vi "IMRP.vi"() -> ()   [LabVIEW 2015]
uses:
  <vilib>/vision/Instrument.llb/Barcode Search Options.ctl
  <vilib>/vision/NI_Vision_Development_Module.lvlib
panel:
  out "String 2":string
  out "String":string
  out "x = y?":bool[](array[boolean])
  out "Barcode Read 2":cluster{"Data":string, "Barcode Type":string}[](array[cluster])
  in  "Delay (s.) 2":dbl(slide)=0.4897959183673469 scale=0.0..2.0
  in  "Stop":bool
  in  "Delay (s.)":dbl(slide)=0.4897959183673469 scale=0.0..2.0
  out "Image":T1(plugin-control)
  out "Number of Barcodes Found":u32
  out "Barcode Read":cluster{"Data":string, "Barcode Type":string}[](array[cluster])
  out "Barcode ANSI/CEN/ISO Grading Report":T2(array[cluster])
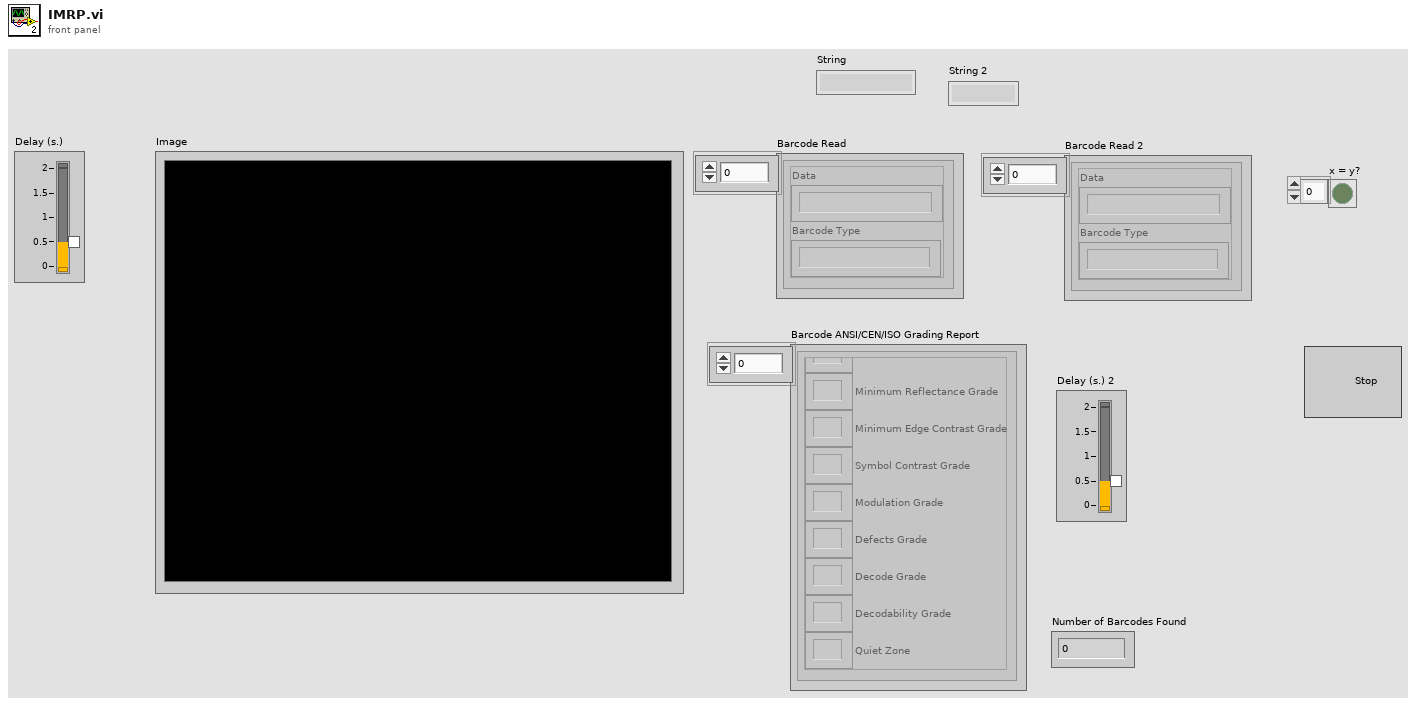
[diagram p1: front panel]
types:
  T1 = typedef "IMAQ Image.ctl" = refnum<image>
  T2 = cluster{"Overall Grade":string, "Edge Determination Grade":string, "Minimum Reflectance Grade":string, "Minimum Edge Contrast Grade":string, "Symbol Contrast Grade":string, "Modulation Grade":string, "Defects Grade":string, "Decode Grade":string, "Decodability Grade":string, "Quiet Zone":string}[]
  T3 = typedef "Barcode Search Options.ctl" = cluster{"Min Bar Width":u32, "Min Edge Strength":u32, "Min Bars":u32, "Skip Location Search?":bool}
  T4 = cluster{"Calculate Grading Report":bool, "Scan Width ":i32}
  T5 = cluster{"Data":string, "Special Char 1":string, "Special Char 2":string, "Checksum(s)":string, "Barcode Type":u32, "Confidence Level":sgl, "Bounding Box":cluster{"x":sgl, "y":sgl}[]}[]
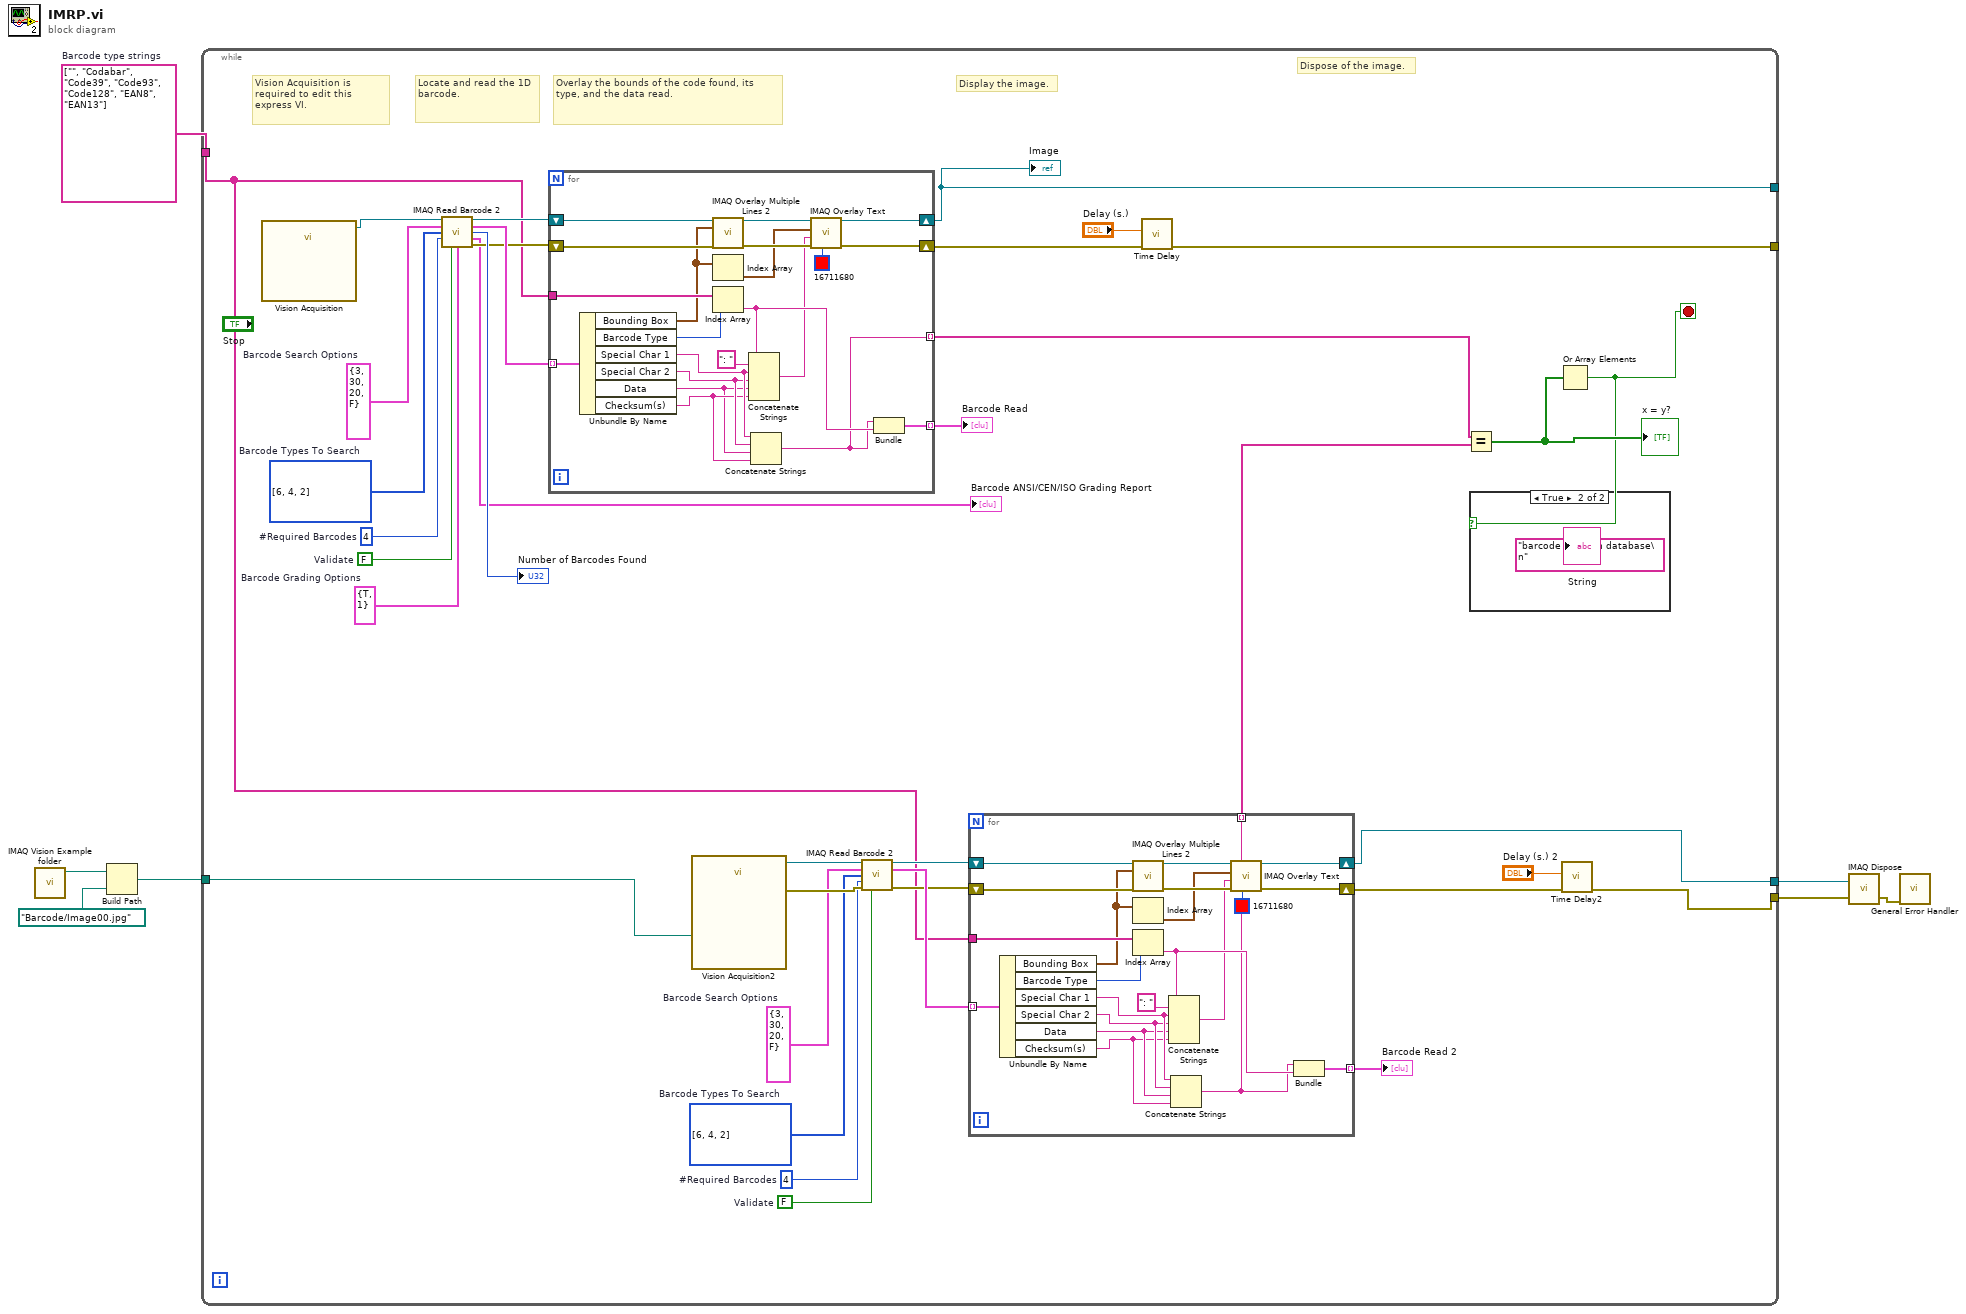
[diagram p0: block diagram]
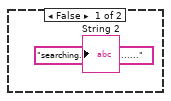
[diagram p2: hidden frame]
diagram:
  w7 = string[] ["", "Codabar", "Code39", "Code93", "Code128", "EAN8", "EAN13"]  # Barcode type strings
  # "Dispose of the image."
  n1 = call "IMAQ Vision Example folder.vi"() -> ("Example Image Path"=w6:path)  [unwired: 11 in]
  n2 = Build Path(base path=w6, name or relative path=path "Barcode/Image00.jpg" ("appended path")) -> (appended path=w4:path)
  n3 = while {
    tunnel: [w35] -> _
    tunnel: [w29] -> _
    tunnel: w7 -> [w15]
    tunnel: w4 -> [w14]
    tunnel: [w13] -> w2
    tunnel: [w12] -> w1
    stop <- w8 stop-if-true
    w17 = T3 {"Min Bar Width"=3, "Min Edge Strength"=30, "Min Bars"=20, "Skip Location Search?"=FALSE}  # Barcode Search Options
    w26 = u32 4  # #Required Barcodes
    w22 = u32[] [6, 4, 2] items=["Reserved", "Codabar", "Code 39", "Code 93", "Code 128", "EAN 8", "EAN 13", "Interleaved 2 of 5", "MSI", "UPCA", "Pharmacode", "RSS Limited"]  # Barcode Types To Search
    w18 = FALSE  # Validate
    w32 = T4 {"Calculate Grading Report"=TRUE, "Scan Width "=1}  # Barcode Grading Options
    w33 = T3 {"Min Bar Width"=3, "Min Edge Strength"=30, "Min Bars"=20, "Skip Location Search?"=FALSE}  # Barcode Search Options
    w43 = u32 4  # #Required Barcodes
    w39 = u32[] [6, 4, 2] items=["Reserved", "Codabar", "Code 39", "Code 93", "Code 128", "EAN 8", "EAN 13", "Interleaved 2 of 5", "MSI", "UPCA", "Pharmacode", "RSS Limited"]  # Barcode Types To Search
    w34 = FALSE  # Validate
    # "Display the image."
    # "Locate and read the 1D barcode."
    # "Vision Acquisition is required to edit this express VI."
    # "Overlay the bounds of the code found, its type, and the data read."
    n4 = call "Vision Acquisition"() -> ("Image Out"=w28:T1)  [unwired: 26 in, 1 out]
    n5 = call "IMAQ Read Barcode 2"("Image"=w28, "Barcode Search Options"=w33, "Barcode Types To Search"=w39, "Num of Required Barcodes"=w43, "Validate"=w34, "Barcode Grading Options"=w32) -> ("Image (duplicate)"=w41:T1, "Barcodes"=w42:T5, "Num of Barcodes"=→"Number of Barcodes Found":u32, "Barcode ANSI/CEN/ISO Grading Report"=→"Barcode ANSI/CEN/ISO Grading Report":T2, "error out"=w38:errorcluster)  [unwired: 5 in]
    n6 = for {
      tunnel: w42 -> [w87] mode=indexing
      tunnel: w15 -> [w86]
      shift-right: [w82] -> w35
      shift-left: w41 -> [w78]
      shift-right: [w79] -> w37
      shift-left: w38 -> [w81]
      tunnel: [w74] -> w31 mode=indexing
      tunnel: [w67] -> w11 mode=indexing
      n7 = Unbundle By Name(w87) -> ("Bounding Box"=w77:cluster{"x":sgl, "y":sgl}[], "Barcode Type"=w75:u32, "Special Char 1"=w71:string, "Special Char 2"=w70:string, "Data"=w68:string, "Checksum(s)"=w69:string)
      n8 = call "IMAQ Overlay Multiple Lines 2"("Image"=w78, "Line End Points"=w77, "error in (no error)"=w81) -> ("Image Out"=w84:T1, "error out"=w80:errorcluster)  [unwired: 11 in]
      n9 = Index Array(array=w77) -> (element=w76:cluster{"x":sgl, "y":sgl})  [unwired: 1 in]
      n10 = Index Array(array=w86, index=w75) -> (element=w73:string)
      n11 = Concatenate Strings(w73, ": " ("string"), w71, w70, w68, w69) -> (w72:string)
      n12 = Concatenate Strings(w71, w70, w68, w69) -> (w67:string)
      n13 = call "IMAQ Overlay Text"("Text Color (black)"=u32 16711680, "error in (no error)"=w80, "String"=w72, "Origin"=w76, "Image"=w84) -> ("error out"=w79:errorcluster, "Image Out"=w82:T1)  [unwired: 5 in]
      n14 = Bundle(w67, w73) -> (w74:cluster{string, string})  [unwired: 1 in]
    }
    "Image" <- w35
    "Barcode Read" <- w31
    n15 = call "Vision Acquisition2"("Image Path"=w14) -> ("Image Out"=w23:T1, "error out"=w27:errorcluster)  [unwired: 24 in, 1 out]
    n16 = call "IMAQ Read Barcode 2"("Image"=w23, "Barcode Search Options"=w17, "Barcode Types To Search"=w22, "Num of Required Barcodes"=w26, "error in (no error)"=w27, "Validate"=w18) -> ("Image (duplicate)"=w24:T1, "Barcodes"=w25:T5, "error out"=w21:errorcluster)  [unwired: 5 in, 2 out]
    n17 = for {
      tunnel: w25 -> [w66] mode=indexing
      tunnel: w15 -> [w65]
      shift-right: [w61] -> w13
      shift-left: w24 -> [w57]
      shift-right: [w58] -> w20
      shift-left: w21 -> [w60]
      tunnel: [w53] -> w16 mode=indexing
      tunnel: [w46] -> w10 mode=indexing
      n18 = Unbundle By Name(w66) -> ("Bounding Box"=w56:cluster{"x":sgl, "y":sgl}[], "Barcode Type"=w54:u32, "Special Char 1"=w50:string, "Special Char 2"=w49:string, "Data"=w48:string, "Checksum(s)"=w47:string)
      n19 = call "IMAQ Overlay Multiple Lines 2"("Image"=w57, "Line End Points"=w56, "error in (no error)"=w60) -> ("Image Out"=w63:T1, "error out"=w59:errorcluster)  [unwired: 11 in]
      n20 = Index Array(array=w56) -> (element=w55:cluster{"x":sgl, "y":sgl})  [unwired: 1 in]
      n21 = Index Array(array=w65, index=w54) -> (element=w52:string)
      n22 = Concatenate Strings(w52, ": " ("string"), w50, w49, w48, w47) -> (w51:string)
      n23 = Concatenate Strings(w50, w49, w48, w47) -> (w46:string)
      n24 = call "IMAQ Overlay Text"("Text Color (black)"=u32 16711680, "error in (no error)"=w59, "String"=w51, "Origin"=w55, "Image"=w63) -> ("error out"=w58:errorcluster, "Image Out"=w61:T1)  [unwired: 5 in]
      n25 = Bundle(w46, w52) -> (w53:cluster{string, string})  [unwired: 1 in]
    }
    "Barcode Read 2" <- w16
    n26 = call "Time Delay"("error in (no error)"=w37, "Delay Time (s)"="Delay (s.)") -> ("error out"=w29:errorcluster)  [unwired: 9 in]
    n27 = Equal?(x=w11, y=w10) -> (x = y?=w9:bool[])
    "x = y?" <- w9
    n28 = Or Array Elements(Boolean array=w9) -> (logical OR=w8:bool)
    n29 = case shown="True" w8 {
      frame False {
        "String 2" <- "searching...................."
      }
      frame True {
        "String" <- "barcode found in database\n"
      }
    }
    n30 = call "Time Delay2"("error in (no error)"=w20, "Delay Time (s)"="Delay (s.) 2") -> ("error out"=w12:errorcluster)  [unwired: 9 in]
  }
  n31 = call "IMAQ Dispose"("Image"=w2, "error in (no error)"=w1) -> ("error out"=w3:errorcluster)  [unwired: 1 in, 3 out]
  n32 = call <vilib>:"General Error Handler.vi"("error in (no error)"=w3) -> ()  [unwired: 10 in, 5 out]
